vi "lxw strerror.vi"(8 "error in (no error)":errorcluster, 11 "error_num":T1 items=["LXW_NO_ERROR"=0, "LXW_ERROR_MEMORY_MALLOC_FAILED"=1, "LXW_ERROR_CREATING_XLSX_FILE"=2, "LXW_ERROR_CREATING_TMPFILE"=3, "LXW_ERROR_READING_TMPFILE"=4, "LXW_ERROR_ZIP_FILE_OPERATION"=5, "LXW_ERROR_ZIP_PARAMETER_ERROR"=6, "LXW_ERROR_ZIP_BAD_ZIP_FILE"=7, "LXW_ERROR_ZIP_INTERNAL_ERROR"=8, "LXW_ERROR_ZIP_FILE_ADD"=9, "LXW_ERROR_ZIP_CLOSE"=10, "LXW_ERROR_FEATURE_NOT_SUPPORTED"=11, "LXW_ERROR_NULL_PARAMETER_IGNORED"=12, "LXW_ERROR_PARAMETER_VALIDATION"=13, "LXW_ERROR_WORKSHEET_INDEX_OUT_OF_RANGE"=20]) -> (0 "error out":errorcluster, 3 "function return":string)   [LabVIEW 2015, in "xlsxwriter.lvlib"]
doc: "const char* lxw_strerror(lxw_error error_num);"
uses:
  xlsxwriter.lvlib
  Controls/lxw_error.ctl
  xlsxwriter.dll
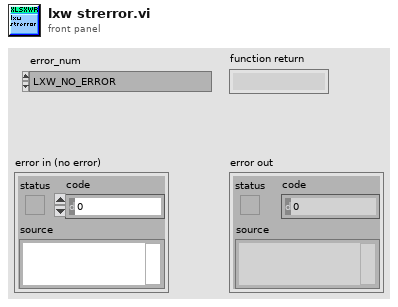
[diagram p1: front panel]
types:
  T1 = typedef "lxw_error.ctl" = u32
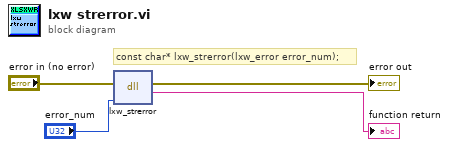
[diagram p0: block diagram]
diagram:
  # "const char* lxw_strerror(lxw_error error_num);"
  n1 = dll-call lib="C:/Users/WDAGUtilityAccount/Desktop/Labview_Example-win32/xlsxwriter.*" fn="lxw_strerror"(error in="error in (no error)", "error_num"="error_num") -> (error out=→"error out":errorcluster, →"function return":string)  [unwired: 3 in, 1 out]
